vi "VCI_InitCan.vi"(8 "VCI_INIT_CONFIG_IN":T1={"AccCode"=0, "AccMask"=4294967295, "Reserved"=0, "Filter"=1, "Timing0"=0, "Timing1"=20, "Mode"=0} {"Timing1" format="%x"; "Timing0" format="%x"; "AccMask" format="%x"}, 9 "CanIndex_IN":u32, 10 "DevIndex_IN":u32, 11 "DevType_IN":u32) -> (1 "CanIndex_OUT":u32, 2 "DevIndex_OUT":u32, 3 "DevType_OUT":u32, 5 "InitCAN_Success?":u32)   [LabVIEW 2014]
uses:
  ControlCAN.dll
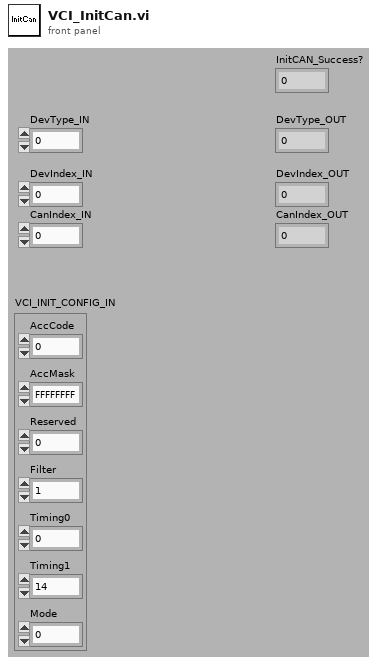
[diagram p1: front panel]
types:
  T1 = cluster{"AccCode":u32, "AccMask":u32, "Reserved":u32, "Filter":u8, "Timing0":u8, "Timing1":u8, "Mode":u8}
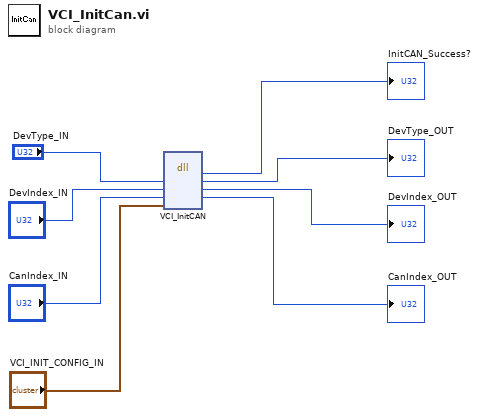
[diagram p0: block diagram]
diagram:
  n1 = dll-call lib="PTH22abs D\tDocuments\tCan总线canControlCAN.dll" fn="VCI_InitCAN"("DevType"="DevType_IN", "DevIndex"="DevIndex_IN", "CanIndex"="CanIndex_IN", "pInit_Config"="VCI_INIT_CONFIG_IN") -> ("InitCan_Success?"=→"InitCAN_Success?":u32, "DevType"=→"DevType_OUT":u32, "DevIndex"=→"DevIndex_OUT":u32, "CanIndex"=→"CanIndex_OUT":u32)  [unwired: 4 in, 2 out]
